vi "GlobalGetConfigurationStatus.vi"() -> ()   [LabVIEW 2013]
panel:
  out "ConfigurationStatus":bool
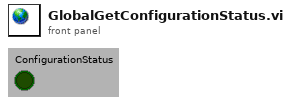
[diagram p1: front panel]
diagram:
